vi "Set Possible Connections.vi"(8 "error in (no error)":errorcluster, 10 "Possible Connections":T1[](array[typedef]), 11 "Hardware Ref in":T2 format="%.0x") -> (0 "error out":errorcluster, 3 "Hardware Ref out":T2 format="%.0x")   [LabVIEW 2017, in "Routing and Faulting Hardware API.lvlib"]
uses:
  Routing and Faulting Hardware API.lvlib
  <vilib>/NI Veristand/Custom Device API/Custom Device Item Ref.ctl
  Types/Possible Connections for Endpoint.ctl
  NationalInstruments.VeriStand.SystemDefinitionAPI
  Routing and Faulting Hardware API Constants.vi
  <vilib>/NI Veristand/Custom Device API/Custom Device API.lvlib
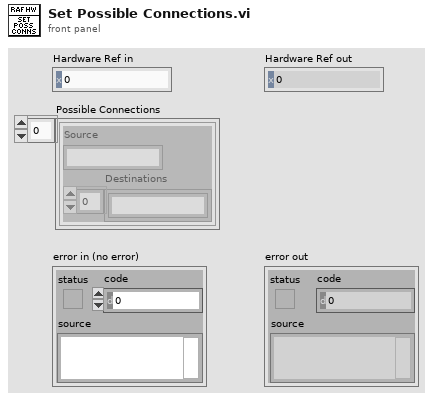
[diagram p1: front panel]
types:
  T1 = typedef "Routing and Faulting Hardware API.lvlib/Possible Connections for Endpoint.ctl" = cluster{"Source":string, "Destinations":string[]}
  T2 = typedef "Custom Device API.lvlib/Custom Device Item Ref.ctl" = u64
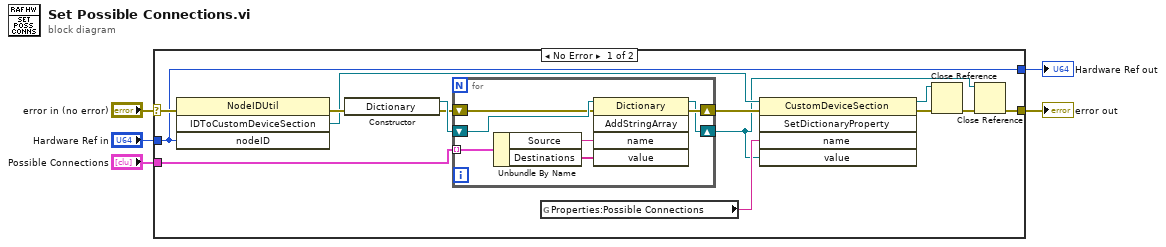
[diagram p0: block diagram]
diagram:
  n1 = case shown="No Error" "error in (no error)" {
    selector: "error in (no error)" -> [w13 w28]
    tunnel: [w7 w28] -> w5
    tunnel: "Hardware Ref in" -> [w12 w27]
    tunnel: [w12 w27] -> w2
    tunnel: "Possible Connections" -> [w11 _]
    frame No Error {
      n2 = invoke class="NodeIDUtil" method="IDToCustomDeviceSection"(error in=w13, "nodeID"=w12) -> (error out=w19:errorcluster, "IDToCustomDeviceSection"=w15:refnum<k24>)  [unwired: 2 in, 2 out]
      n3 = constructor class="Dictionary"(error in=w19) -> (reference out=w18:refnum<k24>, error out=w17:errorcluster)  [unwired: 2 in, 1 out]
      n4 = for {
        shift-right: [w24] -> w16
        shift-left: w17 -> [w25]
        shift-right: [w23] -> w6
        shift-left: w18 -> [w26]
        tunnel: w11 -> [w20] mode=indexing
        n5 = Unbundle By Name(w20) -> ("Source"=w22:string, "Destinations"=w21:string[])
        n6 = invoke class="Dictionary" method="AddStringArray"(reference=w26, error in=w25, "name"=w22, "value"=w21) -> (reference out=w23:refnum<k24>, error out=w24:errorcluster)  [unwired: 1 in, 3 out]
      }
      n7 = global read "Routing and Faulting Hardware API Constants.vi" "Properties:Possible Connections"() -> (w14:string)
      n8 = invoke class="CustomDeviceSection" method="SetDictionaryProperty"(reference=w15, error in=w16, "name"=w14, "value"=w6) -> (reference out=w9:refnum<k24>, error out=w10:errorcluster)  [unwired: 1 in, 3 out]
      n9 = Close Reference(reference=w9, error in (no error)=w10) -> (error out=w8:errorcluster)
      n10 = Close Reference(reference=w6, error in (no error)=w8) -> (error out=w7:errorcluster)
    }
    frame Error {
    }
  }
  "Hardware Ref out" <- w2
  "error out" <- w5
